vi "PAS Functional Test.vi"(8 "error in (no error)":errorcluster, 11 "Test Configuration":T1) -> (0 "Error Out":errorcluster, 3 "Go on?":bool)   [LabVIEW 2015]
uses:
  Controls/Test Configuration.ctl
  Controls/Vacuum Test.ctl
  Controls/Test Timing.ctl
  Controls/Vaccum Thresholds.ctl
  Controls/Helium Test.ctl
  Controls/Helium Thresholds.ctl
  Controls/Functional Test.ctl
  CAN Communication/PAS/PAS.lvclass
panel:
  in  "Quit?":bool
  in  "Abort":bool
  in  "Test":i32(listbox)
  # "PAS Functional Test"
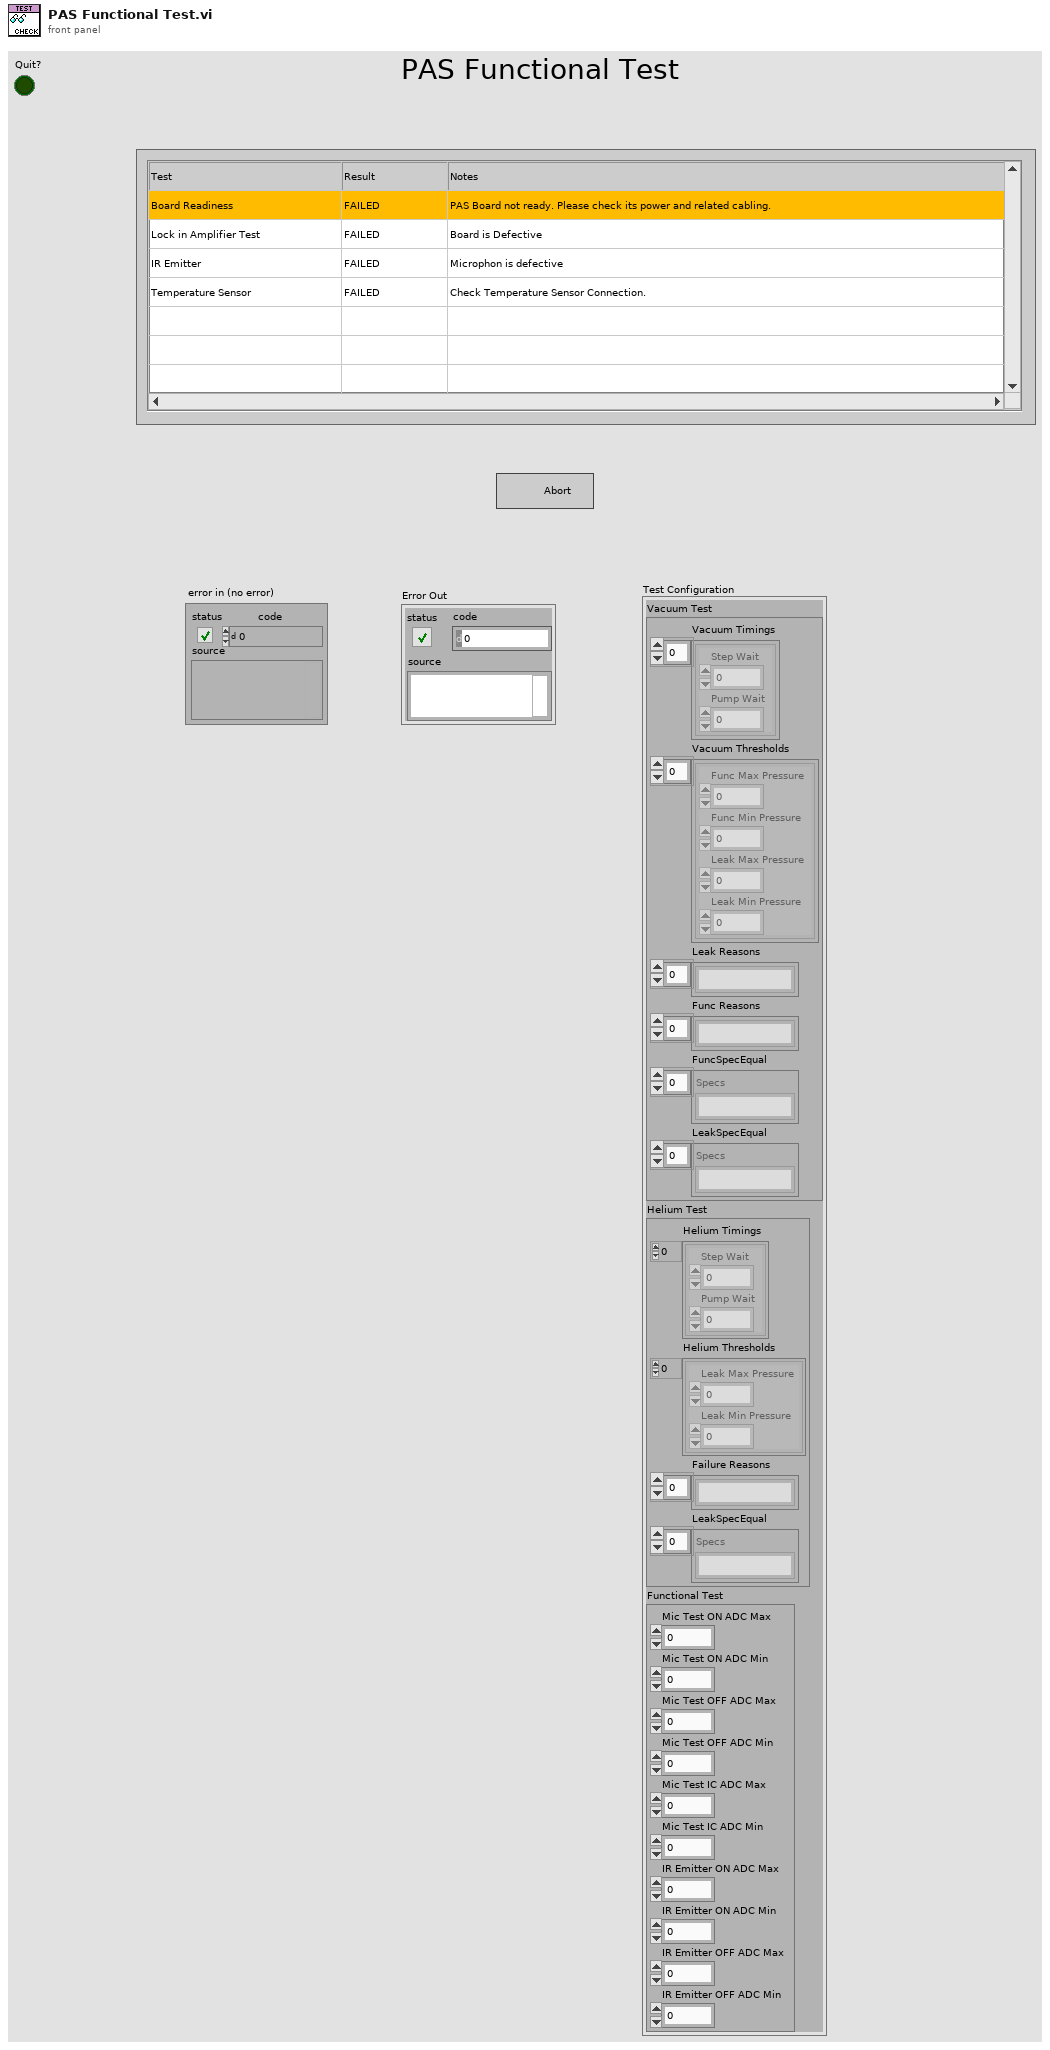
[diagram p1: front panel]
types:
  T1 = typedef "Test Configuration.ctl" = cluster{"Vacuum Test":T2, "Helium Test":T5, "Functional Test":T7}
  T2 = typedef "Vacuum Test.ctl" = cluster{"Vacuum Timings":T3[], "Vacuum Thresholds":T4[], "Leak Reasons":string[], "Func Reasons":string[], "FuncSpecEqual":string[], "LeakSpecEqual":string[]}
  T3 = typedef "Test Timing.ctl" = cluster{"Step Wait":dbl, "Pump Wait":dbl}
  T4 = typedef "Vaccum Thresholds.ctl" = cluster{"Func Max Pressure":dbl, "Func Min Pressure":dbl, "Leak Max Pressure":dbl, "Leak Min Pressure":dbl}
  T5 = typedef "Helium Test.ctl" = cluster{"Helium Timings":T3[], "Helium Thresholds":T6[], "Failure Reasons":string[], "LeakSpecEqual":string[]}
  T6 = typedef "Helium Thresholds.ctl" = cluster{"Leak Max Pressure":dbl, "Leak Min Pressure":dbl}
  T7 = typedef "Functional Test.ctl" = cluster{"Mic Test ON ADC Max":dbl, "Mic Test ON ADC Min":dbl, "Mic Test OFF ADC Max":dbl, "Mic Test OFF ADC Min":dbl, "Mic Test IC ADC Max":dbl, "Mic Test IC ADC Min":dbl, "IR Emitter ON ADC Max":dbl, "IR Emitter ON ADC Min":dbl, "IR Emitter OFF ADC Max":dbl, "IR Emitter OFF ADC Min":dbl}
  T8 = typedef "PAS.lvclass/Session Handle.ctl" = refnum<data-value>
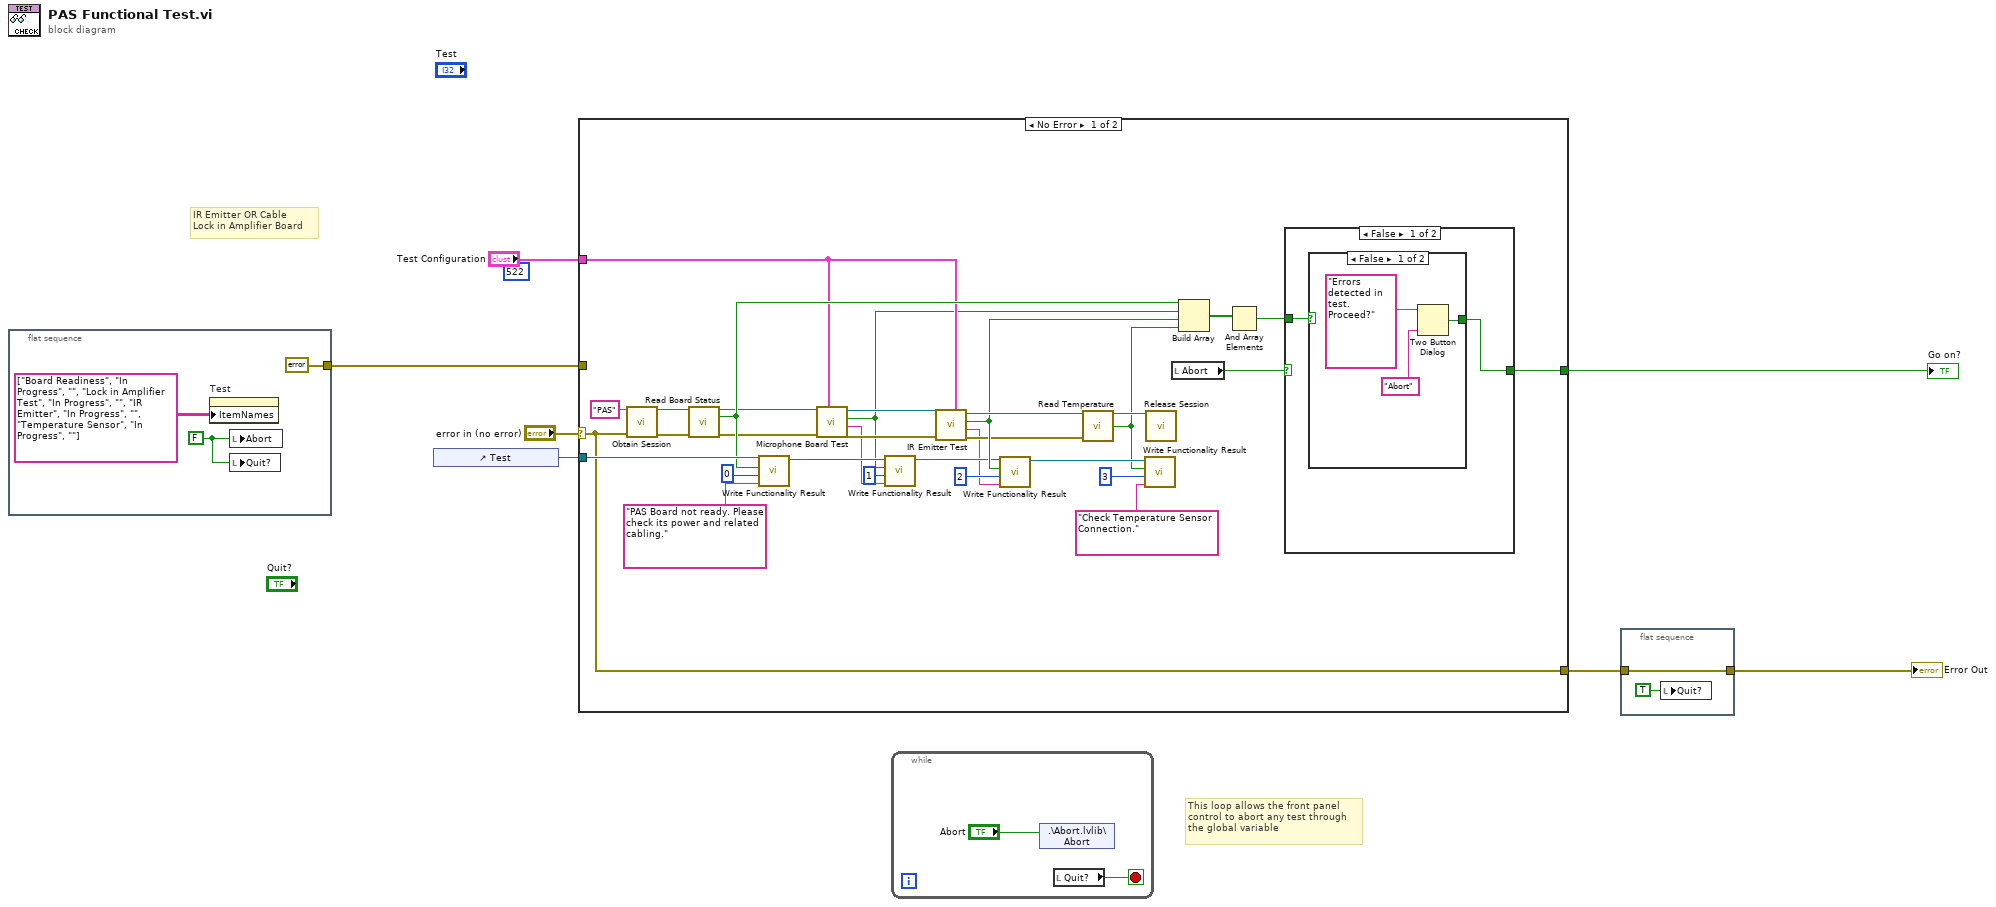
[diagram p0: block diagram]
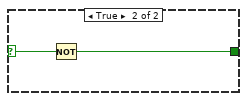
[diagram p3: hidden frame]
diagram:
  (unwired) u16 522 ("identifier")
  # "This loop allows the front panel\ncontrol to abort any test through\nthe global variable"
  # "IR Emitter OR Cable\nLock in Amplifier Board"
  n1 = flat-sequence {
    tunnel: [errorcluster {"status"=FALSE, "code"=0, "source"=""} ("error in (no error)")] -> w6
    frame #0 {
      w8 = FALSE ("Abort")
      n2 = property on="Test" class="MCListbox (strict)"("ItemNames"=string[][] [["Board Readiness", "In Progress", ""], ["Lock in Amplifier Test", "In Progress", ""], ["IR Emitter", "In Progress", ""], ["Temperature Sensor", "In Progress", ""]] ("initialized array")) -> ()  [unwired: 2 in, 2 out]
      n3 = local write "Abort"(w8) -> ()
      n4 = local write "Quit?"(w8) -> ()
    }
  }
  n5 = control-ref of="Test"() -> (w7:refnum<vi>)
  n6 = case shown="No Error" "error in (no error)" {
    selector: "error in (no error)" -> [w28 w51]
    tunnel: w7 -> [w41 _]
    tunnel: w6 -> [_ _]
    tunnel: [w29 _] -> w4
    tunnel: [w28 w51] -> w2
    tunnel: "Test Configuration" -> [w22 _]
    frame No Error {
      n7 = call "Obtain Session.vi"("Session  Name ()"="PAS", "error in (no error)"=w28) -> ("Session Handle"=w11:T8, "error out"=w12:errorcluster)  [unwired: 12 in]
      n8 = call "Read Board Status.vi"("Session Handle in"=w11, "error in (no error)"=w12) -> ("Session Handle out"=w24:T8, "Ready?"=w34:bool, "error out"=w23:errorcluster)  [unwired: 11 in]
      n9 = call "Write Functionality Result.vi"("Reason"="PAS Board not ready. Please check its power and related cabling." ("t"), "Row"=0, "Passed?"=w34, "Reference In"=w41) -> ("Reference Out"=w21:refnum<vi>)  [unwired: 7 in]
      n10 = call "Microphone Board Test.vi"("Test Configuration"=w22, "error in (no error)"=w23, "Session Handle in"=w24) -> ("error out"=w19:errorcluster, "Failure Reason"=w18:string, "Success?"=w16:bool, "Session Handle out"=w20:T8)  [unwired: 5 in]
      n11 = call "Write Functionality Result.vi"("Reason"=w18, "Row"=1, "Passed?"=w16, "Reference In"=w21) -> ("Reference Out"=w15:refnum<vi>)  [unwired: 7 in]
      n12 = call "IR Emitter Test.vi"("Test Configuration"=w22, "error in (no error)"=w19, "Session Handle in"=w20) -> ("error out"=w14:errorcluster, "Failure Reason"=w13:string, "Passed?"=w33:bool, "Session Handle out"=w37:T8)  [unwired: 5 in]
      n13 = call "Write Functionality Result.vi"("Reason"=w13, "Row"=2, "Passed?"=w33, "Reference In"=w15) -> ("Reference Out"=w36:refnum<vi>)  [unwired: 7 in]
      n14 = call "Read Temperature.vi"("Session Handle in"=w37, "error in (no error)"=w14) -> ("Session Handle out"=w35:T8, "Success?"=w32:bool)  [unwired: 9 in, 3 out]
      n15 = call "Write Functionality Result.vi"("Reason"="Check Temperature Sensor Connection." ("t"), "Row"=3, "Passed?"=w32, "Reference In"=w36) -> ()  [unwired: 7 in, 1 out]
      n16 = call "Release Session.vi"("Session Handle"=w35) -> ()  [unwired: 14 in, 1 out]
      n17 = local read "Abort"() -> (w30:bool)
      n18 = Build Array(w34, w16, w33, w32) -> (w31:bool[])
      n19 = And Array Elements(Boolean array=w31) -> (logical AND=w27:bool)
      n20 = case shown="False" w30 {
        selector: w30 -> [_ w50]
        tunnel: [w43 w49] -> w29
        tunnel: w27 -> [w44 _]
        frame False {
          n21 = case shown="False" w44 {
            selector: w44 -> [_ w48]
            tunnel: [w47 w48] -> w43
            frame False {
              n22 = Two Button Dialog(message="Errors detected in test. Proceed?", 1:"Abort" ("F button name (\"Cancel\")")) -> (T button?=w47:bool)  [unwired: 1 in]
            }
            frame True {
            }
          }
        }
        frame True {
          n23 = Not(x=w50) -> (.not. x?=w49:bool)
        }
      }
    }
    frame Error {
    }
  }
  "Go on?" <- w4
  n24 = while {
    stop <- w52 stop-if-true
    n25 = shared-variable ".\\Abort.lvlib\\Abort"("Abort") -> ()  [unwired: 1 in, 1 out]
    n26 = local read "Quit?"() -> (w52:bool)
  }
  n27 = flat-sequence {
    tunnel: w2 -> [w55]
    tunnel: [w55] -> w1
    frame #0 {
      n28 = local write "Quit?"(TRUE ("Quit?")) -> ()
    }
  }
  "Error Out" <- w1
